vi "GetTunnelTerminals.vi"(5 "Tunnel in":refnum<class "Tunnel.lvclass">, 6 "error in":errorcluster, 9 "VI Interpreter in":refnum<class "VI Interpreter.lvclass">) -> (0 "error out":errorcluster, 3 "VI Interpreter out":refnum<class "VI Interpreter.lvclass">, 4 "Tunnel out":refnum<class "Tunnel.lvclass">)   [LabVIEW 2014, in "Raspberry Pi Compatible Compiler for LabVIEW.lvlib" / "VI Interpreter.lvclass"]
uses:
  VI Interpreter.lvclass
  Tunnel/Tunnel.lvclass
  Tunnel/Tunnel.lvclass/Tunnel.ctl
  Terminal/Terminal.lvclass
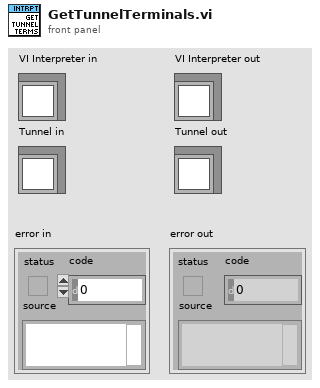
[diagram p1: front panel]
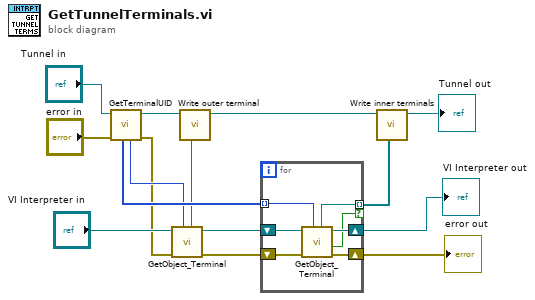
[diagram p0: block diagram]
diagram:
  n1 = call "GetTerminalUID.vi"("error in"="error in", "Tunnel in"="Tunnel in") -> ("error out"=w1:errorcluster, "Tunnel out"=w5:refnum<class "Tunnel.lvclass">, "outer terminal UID"=w10:i32, "inner terminal UIDs"=w12:i32[])  [unwired: 4 in]
  n2 = call "GetObject_Terminal.vi"("UID"=w10, "error in"=w1, "VI Interpreter in"="VI Interpreter in") -> ("error out"=w6:errorcluster, "VI Interpreter out"=w8:refnum<class "VI Interpreter.lvclass">, "Terminal"=w3:refnum<class "Terminal.lvclass">)  [unwired: 3 in, 1 out]
  n3 = call "Write outer terminal.vi"("outer terminal"=w3, "Tunnel in"=w5) -> ("Tunnel out"=w4:refnum<class "Tunnel.lvclass">)  [unwired: 7 in]
  n4 = for {
    shift-right: [w18] -> w15
    shift-left: w8 -> [w22]
    tunnel: w12 -> [w21] mode=indexing
    shift-right: [w20] -> w14
    shift-left: w6 -> [w19]
    tunnel: [w17] -> w11 mode=indexing if=w16
    n5 = call "GetObject_Terminal.vi"("UID"=w21, "error in"=w19, "VI Interpreter in"=w22) -> ("error out"=w20:errorcluster, "found"=w16:bool, "VI Interpreter out"=w18:refnum<class "VI Interpreter.lvclass">, "Terminal"=w17:refnum<class "Terminal.lvclass">)  [unwired: 3 in]
  }
  "error out" <- w14
  "VI Interpreter out" <- w15
  n6 = call "Write inner terminals.vi"("inner terminals"=w11, "Tunnel in"=w4) -> ("Tunnel out"=→"Tunnel out":refnum<class "Tunnel.lvclass">)  [unwired: 7 in]
